vi "Scan_Frequency_Range_SAFE.vi"() -> ()   [LabVIEW 2010]
panel:
  out "Error Phase Shift":cluster{dbl[], dbl[]}(graph)
  out "Error Amplitude":cluster{dbl[], dbl[]}(graph)
  out "Phase Shift":cluster{dbl[], dbl[]}(graph)
  out "Amplitude":cluster{dbl[], dbl[]}(graph)
  in  "Wait [s]":dbl
  in  "Stepsize[Hz]":dbl
  in  "Stop Frequency[Hz]":dbl
  in  "Start Frequency [Hz]":dbl
  out "error out":errorcluster
  in  "error in (no error)":errorcluster
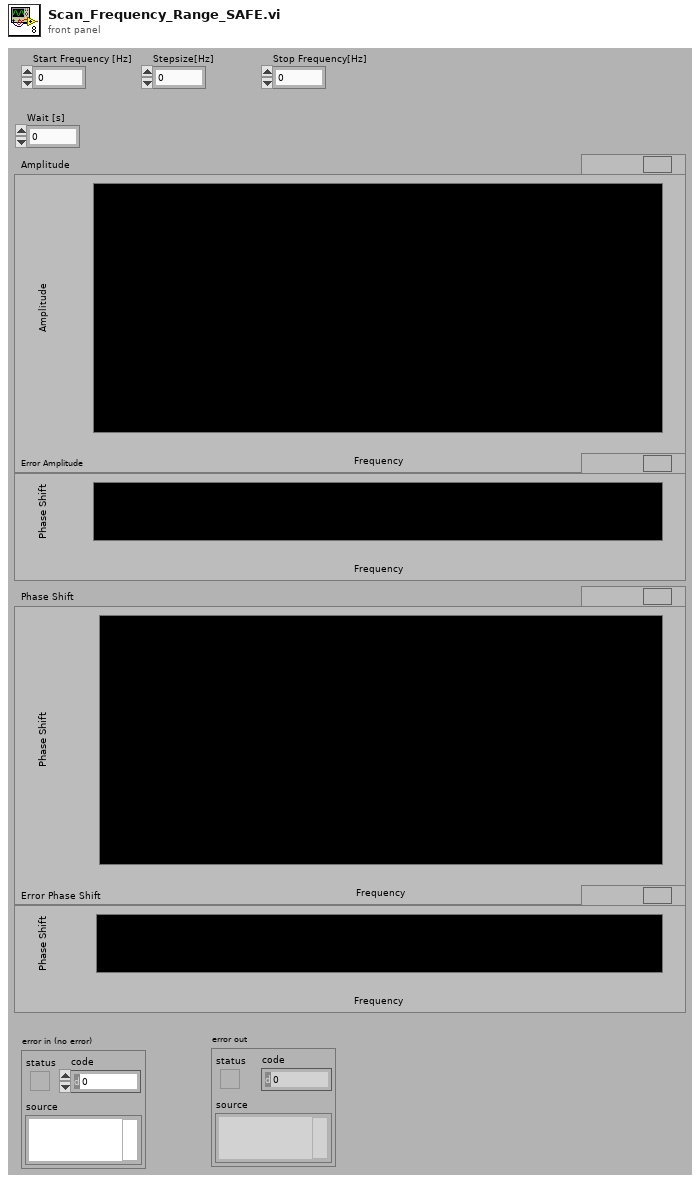
[diagram p1: front panel]
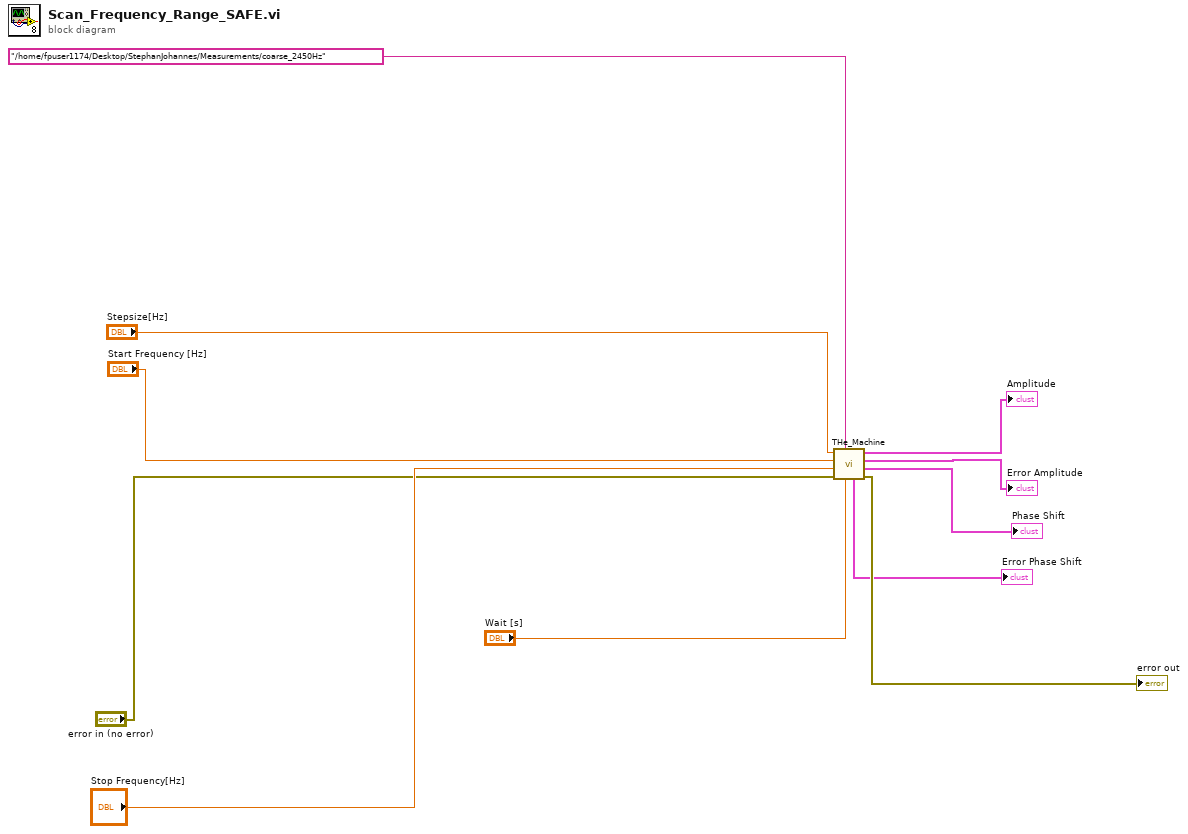
[diagram p0: block diagram]
diagram:
  n1 = call "THe_Machine.vi"("Wait"="Wait [s]", "Adresse"="/home/fpuser1174/Desktop/StephanJohannes/Measurements/coarse_2450Hz", "error in (no error)"="error in (no error)", "Stop Frequency"="Stop Frequency[Hz]", "Start Frequency"="Start Frequency [Hz]", "Stepsize"="Stepsize[Hz]") -> ("error out"=→"error out":errorcluster, "Phase Shift"=→"Phase Shift":cluster{dbl[], dbl[]}, "Error Amplitude"=→"Error Amplitude":cluster{dbl[], dbl[]}, "Amplitude"=→"Amplitude":cluster{dbl[], dbl[]}, "Error Phase Shift"=→"Error Phase Shift":cluster{dbl[], dbl[]})
